vi "ReadData.vi"(8 "error in":errorcluster, 11 "Module Config Selector":i16) -> (0 "error out":errorcluster, 3 "Data Array":sgl[](array[numeric]) format="%.2f")   [LabVIEW 2017, in "BOP_VibAPI_8.lvlib"]
uses:
  <vilib>/addons/InsightCM/Devices/Shared/Cms/Fpga/Acquisition/source/subVIs/VibAPI_8/BOP_VibAPI_8.lvlib
  <vilib>/rvi/eio/common/nirviEmuTemplateMethod_errors.vi
  <vilib>/eio/EIONode/EIONode.xnode
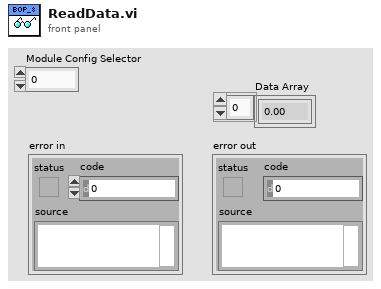
[diagram p1: front panel]
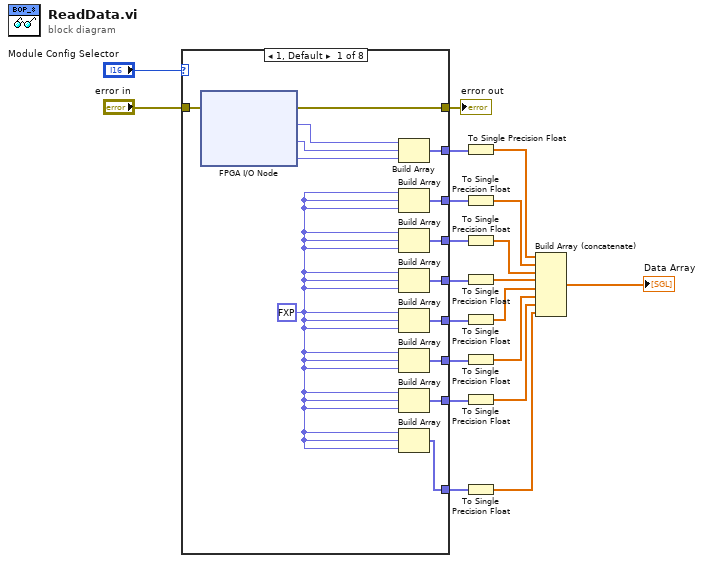
[diagram p0: block diagram]
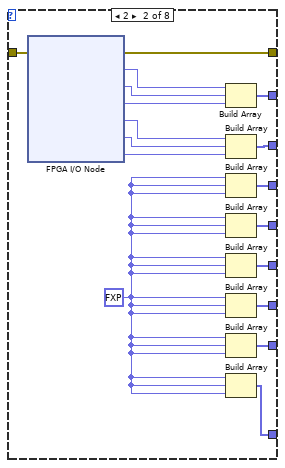
[diagram p2: hidden frame]
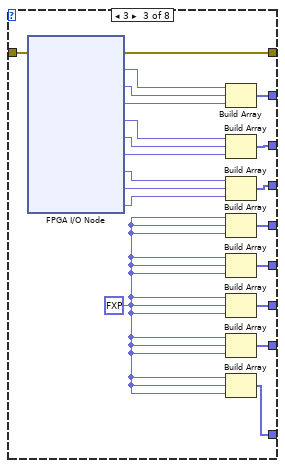
[diagram p3: hidden frame]
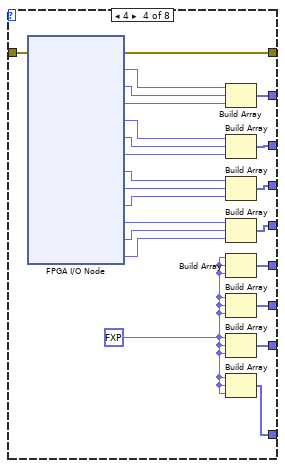
[diagram p4: hidden frame]
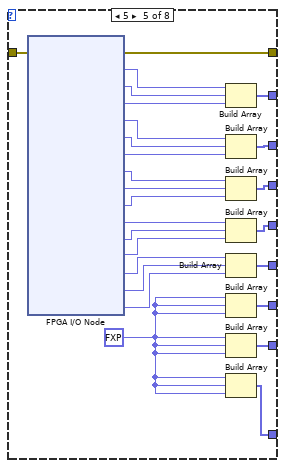
[diagram p5: hidden frame]
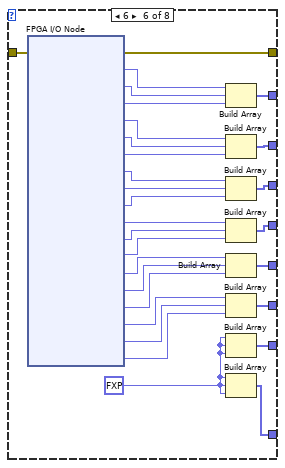
[diagram p6: hidden frame]
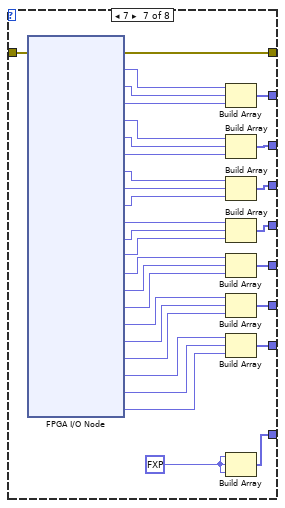
[diagram p7: hidden frame]
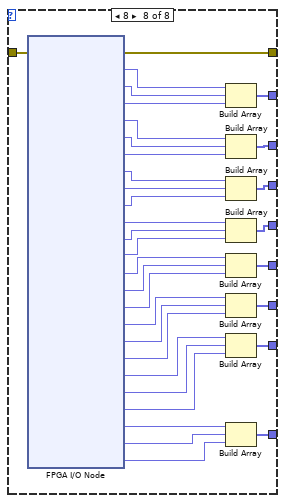
[diagram p8: hidden frame]
diagram:
  n1 = case shown="1, Default" "Module Config Selector" {
    tunnel: "error in" -> [w31 w48 w68 w91 w117 w146 w178 w212]
    tunnel: [w30 w47 w67 w90 w116 w145 w177 w211] -> w19
    tunnel: [w29 w46 w66 w89 w115 w144 w176 w210] -> w16
    tunnel: [w28 w45 w65 w88 w114 w143 w175 w209] -> w14
    tunnel: [w27 w44 w64 w87 w113 w142 w174 w208] -> w12
    tunnel: [w26 w43 w63 w86 w112 w141 w173 w207] -> w10
    tunnel: [w25 w42 w62 w85 w111 w140 w172 w206] -> w8
    tunnel: [w24 w41 w61 w84 w110 w139 w171 w205] -> w6
    tunnel: [w23 w37 w54 w74 w97 w123 w155 w189] -> w4
    tunnel: [w21 w35 w52 w72 w95 w121 w153 w188] -> w2
    frame 1, Default {
      w22 = fxp<+/-,24,7> 0.0 ("Mod1/AI2")
      n2 = xnode "FPGA I/O Node"("error in"=w31) -> ("error out"=w30:errorcluster, "Mod1/AI0"=w32:fxp<+/-,24,7>, "Mod1/AI1"=w34:fxp<+/-,24,7>, "Mod1/AI2"=w33:fxp<+/-,24,7>)  [unwired: 3 in, 3 out]
      n3 = Build Array(w32, w34, w33) -> (w29:fxp<+/-,24,7>[])
      n4 = Build Array(w22, w22, w22) -> (w28:fxp<+/-,24,7>[])
      n5 = Build Array(w22, w22, w22) -> (w27:fxp<+/-,24,7>[])
      n6 = Build Array(w22, w22, w22) -> (w26:fxp<+/-,24,7>[])
      n7 = Build Array(w22, w22, w22) -> (w25:fxp<+/-,24,7>[])
      n8 = Build Array(w22, w22, w22) -> (w24:fxp<+/-,24,7>[])
      n9 = Build Array(w22, w22, w22) -> (w23:fxp<+/-,24,7>[])
      n10 = Build Array(w22, w22, w22) -> (w21:fxp<+/-,24,7>[])
    }
    frame 2 {
      w36 = fxp<+/-,24,7> 0.0 ("Mod1/AI2")
      n11 = xnode "FPGA I/O Node"("error in"=w48) -> ("error out"=w47:errorcluster, "Mod1/AI0"=w49:fxp<+/-,24,7>, "Mod1/AI1"=w51:fxp<+/-,24,7>, "Mod1/AI2"=w50:fxp<+/-,24,7>, "Mod2/AI0"=w40:fxp<+/-,24,7>, "Mod2/AI1"=w39:fxp<+/-,24,7>, "Mod2/AI2"=w38:fxp<+/-,24,7>)  [unwired: 6 in, 6 out]
      n12 = Build Array(w49, w51, w50) -> (w46:fxp<+/-,24,7>[])
      n13 = Build Array(w40, w39, w38) -> (w45:fxp<+/-,24,7>[])
      n14 = Build Array(w36, w36, w36) -> (w44:fxp<+/-,24,7>[])
      n15 = Build Array(w36, w36, w36) -> (w43:fxp<+/-,24,7>[])
      n16 = Build Array(w36, w36, w36) -> (w42:fxp<+/-,24,7>[])
      n17 = Build Array(w36, w36, w36) -> (w41:fxp<+/-,24,7>[])
      n18 = Build Array(w36, w36, w36) -> (w37:fxp<+/-,24,7>[])
      n19 = Build Array(w36, w36, w36) -> (w35:fxp<+/-,24,7>[])
    }
    frame 3 {
      w53 = fxp<+/-,24,7> 0.0 ("Mod1/AI2")
      n20 = xnode "FPGA I/O Node"("error in"=w68) -> ("error out"=w67:errorcluster, "Mod1/AI0"=w69:fxp<+/-,24,7>, "Mod1/AI1"=w71:fxp<+/-,24,7>, "Mod1/AI2"=w70:fxp<+/-,24,7>, "Mod2/AI0"=w60:fxp<+/-,24,7>, "Mod2/AI1"=w59:fxp<+/-,24,7>, "Mod2/AI2"=w58:fxp<+/-,24,7>, "Mod3/AI0"=w57:fxp<+/-,24,7>, "Mod3/AI1"=w56:fxp<+/-,24,7>, "Mod3/AI2"=w55:fxp<+/-,24,7>)  [unwired: 9 in, 9 out]
      n21 = Build Array(w69, w71, w70) -> (w66:fxp<+/-,24,7>[])
      n22 = Build Array(w60, w59, w58) -> (w65:fxp<+/-,24,7>[])
      n23 = Build Array(w57, w56, w55) -> (w64:fxp<+/-,24,7>[])
      n24 = Build Array(w53, w53, w53) -> (w63:fxp<+/-,24,7>[])
      n25 = Build Array(w53, w53, w53) -> (w62:fxp<+/-,24,7>[])
      n26 = Build Array(w53, w53, w53) -> (w61:fxp<+/-,24,7>[])
      n27 = Build Array(w53, w53, w53) -> (w54:fxp<+/-,24,7>[])
      n28 = Build Array(w53, w53, w53) -> (w52:fxp<+/-,24,7>[])
    }
    frame 4 {
      w73 = fxp<+/-,24,7> 0.0 ("Mod1/AI2")
      n29 = xnode "FPGA I/O Node"("error in"=w91) -> ("error out"=w90:errorcluster, "Mod1/AI0"=w92:fxp<+/-,24,7>, "Mod1/AI1"=w94:fxp<+/-,24,7>, "Mod1/AI2"=w93:fxp<+/-,24,7>, "Mod2/AI0"=w83:fxp<+/-,24,7>, "Mod2/AI1"=w82:fxp<+/-,24,7>, "Mod2/AI2"=w81:fxp<+/-,24,7>, "Mod3/AI0"=w80:fxp<+/-,24,7>, "Mod3/AI1"=w79:fxp<+/-,24,7>, "Mod3/AI2"=w78:fxp<+/-,24,7>, "Mod4/AI0"=w77:fxp<+/-,24,7>, "Mod4/AI1"=w76:fxp<+/-,24,7>, "Mod4/AI2"=w75:fxp<+/-,24,7>)  [unwired: 12 in, 12 out]
      n30 = Build Array(w92, w94, w93) -> (w89:fxp<+/-,24,7>[])
      n31 = Build Array(w83, w82, w81) -> (w88:fxp<+/-,24,7>[])
      n32 = Build Array(w80, w79, w78) -> (w87:fxp<+/-,24,7>[])
      n33 = Build Array(w77, w76, w75) -> (w86:fxp<+/-,24,7>[])
      n34 = Build Array(w73, w73, w73) -> (w85:fxp<+/-,24,7>[])
      n35 = Build Array(w73, w73, w73) -> (w84:fxp<+/-,24,7>[])
      n36 = Build Array(w73, w73, w73) -> (w74:fxp<+/-,24,7>[])
      n37 = Build Array(w73, w73, w73) -> (w72:fxp<+/-,24,7>[])
    }
    frame 5 {
      w96 = fxp<+/-,24,7> 0.0 ("Mod1/AI2")
      n38 = xnode "FPGA I/O Node"("error in"=w117) -> ("error out"=w116:errorcluster, "Mod1/AI0"=w118:fxp<+/-,24,7>, "Mod1/AI1"=w120:fxp<+/-,24,7>, "Mod1/AI2"=w119:fxp<+/-,24,7>, "Mod2/AI0"=w109:fxp<+/-,24,7>, "Mod2/AI1"=w108:fxp<+/-,24,7>, "Mod2/AI2"=w107:fxp<+/-,24,7>, "Mod3/AI0"=w106:fxp<+/-,24,7>, "Mod3/AI1"=w105:fxp<+/-,24,7>, "Mod3/AI2"=w104:fxp<+/-,24,7>, "Mod4/AI0"=w103:fxp<+/-,24,7>, "Mod4/AI1"=w102:fxp<+/-,24,7>, "Mod4/AI2"=w101:fxp<+/-,24,7>, "Mod5/AI0"=w100:fxp<+/-,24,7>, "Mod5/AI1"=w99:fxp<+/-,24,7>, "Mod5/AI2"=w98:fxp<+/-,24,7>)  [unwired: 15 in, 15 out]
      n39 = Build Array(w118, w120, w119) -> (w115:fxp<+/-,24,7>[])
      n40 = Build Array(w109, w108, w107) -> (w114:fxp<+/-,24,7>[])
      n41 = Build Array(w106, w105, w104) -> (w113:fxp<+/-,24,7>[])
      n42 = Build Array(w103, w102, w101) -> (w112:fxp<+/-,24,7>[])
      n43 = Build Array(w100, w99, w98) -> (w111:fxp<+/-,24,7>[])
      n44 = Build Array(w96, w96, w96) -> (w110:fxp<+/-,24,7>[])
      n45 = Build Array(w96, w96, w96) -> (w97:fxp<+/-,24,7>[])
      n46 = Build Array(w96, w96, w96) -> (w95:fxp<+/-,24,7>[])
    }
    frame 6 {
      w122 = fxp<+/-,24,7> 0.0 ("Mod1/AI2")
      n47 = xnode "FPGA I/O Node"("error in"=w146) -> ("error out"=w145:errorcluster, "Mod1/AI0"=w147:fxp<+/-,24,7>, "Mod1/AI1"=w149:fxp<+/-,24,7>, "Mod1/AI2"=w148:fxp<+/-,24,7>, "Mod2/AI0"=w138:fxp<+/-,24,7>, "Mod2/AI1"=w137:fxp<+/-,24,7>, "Mod2/AI2"=w136:fxp<+/-,24,7>, "Mod3/AI0"=w135:fxp<+/-,24,7>, "Mod3/AI1"=w134:fxp<+/-,24,7>, "Mod3/AI2"=w133:fxp<+/-,24,7>, "Mod4/AI0"=w132:fxp<+/-,24,7>, "Mod4/AI1"=w131:fxp<+/-,24,7>, "Mod4/AI2"=w130:fxp<+/-,24,7>, "Mod5/AI0"=w129:fxp<+/-,24,7>, "Mod5/AI1"=w128:fxp<+/-,24,7>, "Mod5/AI2"=w127:fxp<+/-,24,7>, "Mod6/AI0"=w126:fxp<+/-,24,7>, "Mod6/AI1"=w125:fxp<+/-,24,7>, "Mod6/AI2"=w124:fxp<+/-,24,7>)  [unwired: 18 in, 18 out]
      n48 = Build Array(w147, w149, w148) -> (w144:fxp<+/-,24,7>[])
      n49 = Build Array(w138, w137, w136) -> (w143:fxp<+/-,24,7>[])
      n50 = Build Array(w135, w134, w133) -> (w142:fxp<+/-,24,7>[])
      n51 = Build Array(w132, w131, w130) -> (w141:fxp<+/-,24,7>[])
      n52 = Build Array(w129, w128, w127) -> (w140:fxp<+/-,24,7>[])
      n53 = Build Array(w126, w125, w124) -> (w139:fxp<+/-,24,7>[])
      n54 = Build Array(w122, w122, w122) -> (w123:fxp<+/-,24,7>[])
      n55 = Build Array(w122, w122, w122) -> (w121:fxp<+/-,24,7>[])
    }
    frame 7 {
      w154 = fxp<+/-,24,7> 0.0 ("Mod1/AI2")
      n56 = xnode "FPGA I/O Node"("error in"=w178) -> ("error out"=w177:errorcluster, "Mod1/AI0"=w179:fxp<+/-,24,7>, "Mod1/AI1"=w181:fxp<+/-,24,7>, "Mod1/AI2"=w180:fxp<+/-,24,7>, "Mod2/AI0"=w170:fxp<+/-,24,7>, "Mod2/AI1"=w169:fxp<+/-,24,7>, "Mod2/AI2"=w168:fxp<+/-,24,7>, "Mod3/AI0"=w167:fxp<+/-,24,7>, "Mod3/AI1"=w166:fxp<+/-,24,7>, "Mod3/AI2"=w165:fxp<+/-,24,7>, "Mod4/AI0"=w164:fxp<+/-,24,7>, "Mod4/AI1"=w163:fxp<+/-,24,7>, "Mod4/AI2"=w162:fxp<+/-,24,7>, "Mod5/AI0"=w161:fxp<+/-,24,7>, "Mod5/AI1"=w160:fxp<+/-,24,7>, "Mod5/AI2"=w159:fxp<+/-,24,7>, "Mod6/AI0"=w158:fxp<+/-,24,7>, "Mod6/AI1"=w157:fxp<+/-,24,7>, "Mod6/AI2"=w156:fxp<+/-,24,7>, "Mod7/AI0"=w152:fxp<+/-,24,7>, "Mod7/AI1"=w151:fxp<+/-,24,7>, "Mod7/AI2"=w150:fxp<+/-,24,7>)  [unwired: 21 in, 21 out]
      n57 = Build Array(w179, w181, w180) -> (w176:fxp<+/-,24,7>[])
      n58 = Build Array(w170, w169, w168) -> (w175:fxp<+/-,24,7>[])
      n59 = Build Array(w167, w166, w165) -> (w174:fxp<+/-,24,7>[])
      n60 = Build Array(w164, w163, w162) -> (w173:fxp<+/-,24,7>[])
      n61 = Build Array(w161, w160, w159) -> (w172:fxp<+/-,24,7>[])
      n62 = Build Array(w158, w157, w156) -> (w171:fxp<+/-,24,7>[])
      n63 = Build Array(w152, w151, w150) -> (w155:fxp<+/-,24,7>[])
      n64 = Build Array(w154, w154, w154) -> (w153:fxp<+/-,24,7>[])
    }
    frame 8 {
      n65 = xnode "FPGA I/O Node"("error in"=w212) -> ("error out"=w211:errorcluster, "Mod1/AI0"=w213:fxp<+/-,24,7>, "Mod1/AI1"=w215:fxp<+/-,24,7>, "Mod1/AI2"=w214:fxp<+/-,24,7>, "Mod2/AI0"=w204:fxp<+/-,24,7>, "Mod2/AI1"=w203:fxp<+/-,24,7>, "Mod2/AI2"=w202:fxp<+/-,24,7>, "Mod3/AI0"=w201:fxp<+/-,24,7>, "Mod3/AI1"=w200:fxp<+/-,24,7>, "Mod3/AI2"=w199:fxp<+/-,24,7>, "Mod4/AI0"=w198:fxp<+/-,24,7>, "Mod4/AI1"=w197:fxp<+/-,24,7>, "Mod4/AI2"=w196:fxp<+/-,24,7>, "Mod5/AI0"=w195:fxp<+/-,24,7>, "Mod5/AI1"=w194:fxp<+/-,24,7>, "Mod5/AI2"=w193:fxp<+/-,24,7>, "Mod6/AI0"=w192:fxp<+/-,24,7>, "Mod6/AI1"=w191:fxp<+/-,24,7>, "Mod6/AI2"=w190:fxp<+/-,24,7>, "Mod7/AI0"=w187:fxp<+/-,24,7>, "Mod7/AI1"=w186:fxp<+/-,24,7>, "Mod7/AI2"=w185:fxp<+/-,24,7>, "Mod8/AI0"=w184:fxp<+/-,24,7>, "Mod8/AI1"=w183:fxp<+/-,24,7>, "Mod8/AI2"=w182:fxp<+/-,24,7>)  [unwired: 24 in, 24 out]
      n66 = Build Array(w213, w215, w214) -> (w210:fxp<+/-,24,7>[])
      n67 = Build Array(w204, w203, w202) -> (w209:fxp<+/-,24,7>[])
      n68 = Build Array(w201, w200, w199) -> (w208:fxp<+/-,24,7>[])
      n69 = Build Array(w198, w197, w196) -> (w207:fxp<+/-,24,7>[])
      n70 = Build Array(w195, w194, w193) -> (w206:fxp<+/-,24,7>[])
      n71 = Build Array(w192, w191, w190) -> (w205:fxp<+/-,24,7>[])
      n72 = Build Array(w187, w186, w185) -> (w189:fxp<+/-,24,7>[])
      n73 = Build Array(w184, w183, w182) -> (w188:fxp<+/-,24,7>[])
    }
  }
  "error out" <- w19
  n74 = To Single Precision Float(number=w16) -> (single precision float=w15:sgl[])
  n75 = To Single Precision Float(number=w14) -> (single precision float=w13:sgl[])
  n76 = To Single Precision Float(number=w12) -> (single precision float=w11:sgl[])
  n77 = To Single Precision Float(number=w10) -> (single precision float=w9:sgl[])
  n78 = To Single Precision Float(number=w8) -> (single precision float=w7:sgl[])
  n79 = To Single Precision Float(number=w6) -> (single precision float=w5:sgl[])
  n80 = To Single Precision Float(number=w4) -> (single precision float=w3:sgl[])
  n81 = To Single Precision Float(number=w2) -> (single precision float=w1:sgl[])
  n82 = Build Array (concatenate)(w15, w13, w11, w9, w7, w5, w3, w1) -> (→"Data Array":sgl[])
